vi "ismatest.vi"() -> ()   [LabVIEW 2016]
uses:
  BERTTA.dll
panel:
  out "return type":dbl
  in  "speed":dbl
  in  "port":i32=6
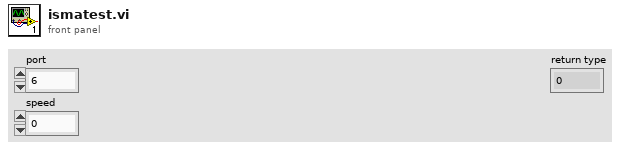
[diagram p1: front panel]
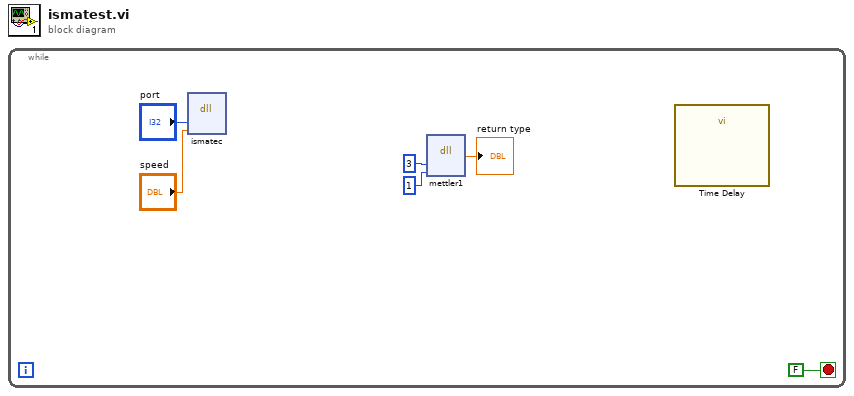
[diagram p0: block diagram]
diagram:
  n1 = while {
    stop <- FALSE stop-if-true
    n2 = dll-call lib="C:/Users/shresplab/OneDrive - Kemira Oyj/Documents/GitHub/Bertta/BERTTA/x64/Debug/BERTTA.dll" fn="ismatec"("port"="port", "speed"="speed") -> ()  [unwired: 6 in, 2 out]
    n3 = dll-call lib="C:/Users/shresplab/OneDrive - Kemira Oyj/Documents/GitHub/Bertta/BERTTA/x64/Debug/BERTTA.dll" fn="mettler1"("port"=3, "msg"=1) -> ("return type"=→"return type":dbl)  [unwired: 5 in, 2 out]
    n4 = call "Time Delay"() -> ()  [unwired: 11 in, 1 out]
  }
